vi "destroyReferences.vi"(8 "error in (no error)":errorcluster, 11 "tcpServerBase in":refnum<class "TcpServerBase.lvclass">) -> (0 "error out":errorcluster, 3 "tcpServerBase out":refnum<class "TcpServerBase.lvclass">)   [LabVIEW 2018, in "TcpServerBase.lvclass"]
doc: "Release notifier references and unregister user event references."
uses:
  TcpServerBase.lvclass
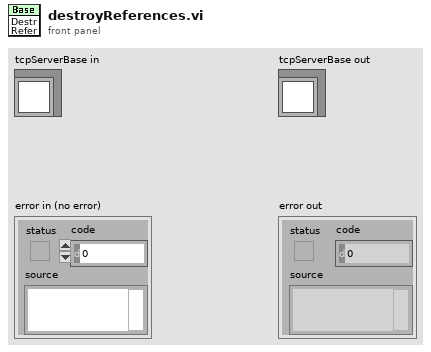
[diagram p1: front panel]
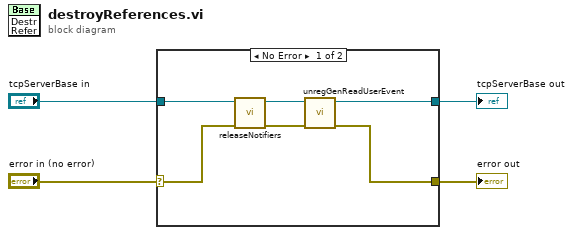
[diagram p0: block diagram]
diagram:
  n1 = case shown="No Error" "error in (no error)" {
    selector: "error in (no error)" -> [w9 w12]
    tunnel: "tcpServerBase in" -> [w10 w11]
    tunnel: [w7 w11] -> w3
    tunnel: [w5 w12] -> w1
    frame No Error {
      n2 = call "releaseNotifiers.vi"("error in (no error)"=w9, "tcpServerBase in"=w10) -> ("error out"=w6:errorcluster, "tcpServerBase out"=w8:refnum<class "TcpServerBase.lvclass">)  [unwired: 8 in]
      n3 = call "unregGenReadUserEvent.vi"("error in (no error)"=w6, "tcpServerBase in"=w8) -> ("error out"=w5:errorcluster, "tcpServerBase out"=w7:refnum<class "TcpServerBase.lvclass">)  [unwired: 8 in]
    }
    frame Error {
    }
  }
  "tcpServerBase out" <- w3
  "error out" <- w1
